vi "After Launch Init Core.vi"(8 "error in (no error)":errorcluster, 11 "CS++OPCUAInterface in":refnum<class "CS++OPCUAInterface.lvclass">) -> (0 "error out":errorcluster, 3 "CS++OPCUAInterface out":refnum<class "CS++OPCUAInterface.lvclass">)   [LabVIEW 2014, in "CS++OPCUAInterface.lvlib" / "CS++OPCUAInterface.lvclass"]
doc: "Launch PVMonitor and register callback messages for specified PV-Write-URLs\n\n\nUse <b>Pre Launch init.vi</b> method only for sanity checks that are supposed to prevent the actor from launching if they fail. Use <B>this</B> method instead to initialize unique resources that must be released during the <b>Stop Core.vi</b> method. A corresponding high priority message will become dispatched before the <B>Actor Framework.lvlib:Actor.lvclass.Actor Core.vi</b> is called.\n\n<b>Derived classed should call the parent methode first</b> and their own initialization code after.\n\nRefer also to the ongoing discussion at https://decibel.ni.com/content/message/57394#57394."
uses:
  CS++OPCUAInterface.lvclass
  CS++OPCUAInterface.lvclass/CS++OPCUAInterface.ctl
  CSPP_Core/Actors/CS++PVMonitor/CS++PVMonitor.lvclass
  CS++OPCUAInterface Messages/Update-PV Msg/Update-PV Msg.lvclass
  CSPP_Core/Classes/CS++ProcessVariables/PVConnection/PVConnection.lvclass/PVConnection.ctl
  CSPP_Core/Actors/CS++PVMonitor Messages/CS++PVUpdate Msg/CS++PVUpdate Msg.lvclass/CS++PVUpdate Msg.ctl
  CSPP_Core/Actors/CS++BaseActor/CS++BaseActor.lvclass/CS++BaseActor.ctl
  <vilib>/ActorFramework/Actor/Actor.lvclass/Actor.ctl
  <vilib>/ActorFramework/Message Enqueuer/Message Enqueuer.lvclass/Message Enqueuer.ctl
  CSPP_Core/Actors/CS++PVMonitor Messages/Register PVs Msg/Register PVs Msg.lvclass/Register PVs Msg.ctl
  <vilib>/ActorFramework/Message Enqueuer/Init from Existing Queue.vi
  <vilib>/ActorFramework/Message Enqueuer/Enqueue.vi
  <vilib>/ActorFramework/Message Priority Queue/Priority Enqueue.vi
  CSPP_Core/Actors/CS++BaseActor/CS++BaseActor.lvclass
  CSPP_Core/Actors/CS++PVMonitor Messages/Register PVs Msg/Register PVs Msg.lvclass
  <vilib>/ActorFramework/Message Enqueuer/Message Enqueuer.lvclass
  CSPP_Core/Classes/CS++BaseClasses/Factory/CS++Factory.lvclass
  CSPP_Core/Classes/CS++ProcessVariables/ProcessVariable/PV.lvclass
  <vilib>/ActorFramework/Actor/Actor.lvclass
  CSPP_Core/Actors/CS++PVMonitor Messages/CS++PVUpdate Msg/CS++PVUpdate Msg.lvclass
  CSPP_Core/Classes/CS++ProcessVariables/PVConnection/PVConnection.lvclass
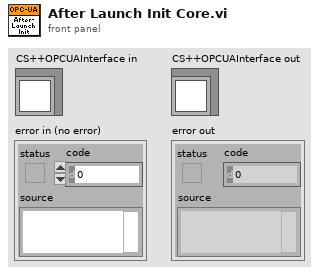
[diagram p1: front panel]
types:
  T1 = cluster{"Self Enqueuer":refnum<class "Message Enqueuer.lvclass">, refnum<class "Update-PV Msg.lvclass">[]}
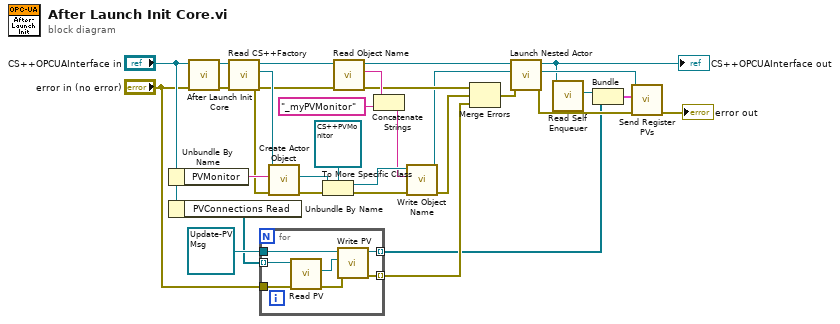
[diagram p0: block diagram]
diagram:
  n1 = Unbundle By Name("CS++OPCUAInterface in") -> ("PVMonitor"=w26:string)
  n2 = Unbundle By Name("CS++OPCUAInterface in") -> ("PVConnections Read"=w10:refnum<class "PVConnection.lvclass">[])
  n3 = call-parent "After Launch Init Core.vi"("error in (no error)"="error in (no error)", "CS++BaseActor in"="CS++OPCUAInterface in") -> ("error out"=w18:errorcluster, "CS++BaseActor out"=w20:refnum<class "CS++OPCUAInterface.lvclass">)  [unwired: 8 in]
  n4 = call "Read CS++Factory.vi"("error in (no error)"=w18, "CS++BaseActor in"=w20) -> ("error out"=w9:errorcluster, "CS++Factory"=w25:refnum<class "CS++Factory.lvclass">, "CS++BaseActor out"=w19:refnum<class "CS++OPCUAInterface.lvclass">)  [unwired: 7 in]
  n5 = for {
    tunnel: refnum<class "Update-PV Msg.lvclass"> refnum ("CS++OPCUAInterface.lvlib:Update-PV Msg.lvclass") -> [w38]
    tunnel: w10 -> [w35] mode=indexing
    tunnel: [w37] -> w5 mode=indexing
    tunnel: [w36] -> w2 mode=indexing
    tunnel: "error in (no error)" -> [w34]
    n6 = call "Read PV.vi"("error in (no error)"=w34, "PVConnection in"=w35) -> ("error out"=w33:errorcluster, "PV"=w32:refnum<class "PV.lvclass">)  [unwired: 7 in, 1 out]
    n7 = call "Write PV.vi"("error in (no error)"=w33, "PV"=w32, "CS++PVUpdate Msg in"=w38) -> ("error out"=w37:errorcluster, "CS++PVUpdate Msg out"=w36:refnum<class "Update-PV Msg.lvclass">)  [unwired: 7 in]
  }
  n8 = call "Create Actor Object.vi"("error in (no error)"=w9, "Object Name"=w26, "CS++Factory in"=w25) -> ("error out"=w28:errorcluster, "CS++BaseActor"=w27:refnum<class "CS++BaseActor.lvclass">)  [unwired: 5 in, 2 out]
  n9 = To More Specific Class(target class=refnum<class "CS++PVMonitor.lvclass"> refnum ("CS++PVMonitor.lvlib:CS++PVMonitor.lvclass"), reference=w27, error in=w28) -> (specific class reference=w24:refnum<class "CS++PVMonitor.lvclass">, error out=w23:errorcluster)
  n10 = call "Read Object Name.vi"("error in (no error)"=w9, "CS++BaseActor in"=w19) -> ("error out"=w30:errorcluster, "Object Name"=w31:string, "CS++BaseActor out"=w13:refnum<class "CS++OPCUAInterface.lvclass">)  [unwired: 7 in]
  n11 = Concatenate Strings(w31, "_myPVMonitor" ("Object Name")) -> (w21:string)
  n12 = call "Write Object Name.vi"("error in (no error)"=w23, "Object Name"=w21, "CS++BaseActor in"=w24) -> ("error out"=w6:errorcluster, "CS++BaseActor out"=w8:refnum<class "CS++PVMonitor.lvclass">)  [unwired: 7 in]
  n13 = Merge Errors(w30, w6, w5) -> (w7:errorcluster)
  n14 = call <vilib>:"Launch Nested Actor.vi"("error in (no error)"=w7, "Nested Actor"=w8, "Caller Actor in"=w13) -> ("error out"=w4:errorcluster, "Nested Actor's Enqueuer"=w17:refnum<class "Message Enqueuer.lvclass">, "Caller Actor out"=w12:refnum<class "CS++OPCUAInterface.lvclass">)  [unwired: 6 in]
  "CS++OPCUAInterface out" <- w12
  n15 = call <vilib>:"Read Self Enqueuer.vi"("Actor"=w12) -> ("Self Enqueuer"=w15:refnum<class "Message Enqueuer.lvclass">)  [unwired: 10 in]
  n16 = Bundle("Self Enqueuer"=w15, w2) -> (w16:T1)  [unwired: 1 in]
  n17 = call "Send Register PVs.vi"("error in (no error)"=w4, "Register Info"=w16, "Message Enqueuer"=w17) -> ("error out"=→"error out":errorcluster)  [unwired: 7 in, 1 out]
